vi "ListAllElementsDC.vi"(8 "error in (no error)":errorcluster, 11 "DataCollector in":refnum<class "DataCollector.lvclass">) -> (0 "error out":errorcluster, 1 "List of Fieldelements":string[](array[string]), 2 "Energy System Setup":string[][](table) caption="Result Set (from first statement with results)", 3 "DataCollector out":refnum<class "DataCollector.lvclass">)   [LabVIEW 2017, in "DataCollector.lvclass"]
uses:
  DataCollector.lvclass
  DataCollector.lvclass/DataCollector.ctl
  <vilib>/drjdpowell/SQLite Library/SQL Connection/Execute SQL.vi
  <vilib>/drjdpowell/SQLite Library/SQLite.lvlib
  <vilib>/drjdpowell/SQLite Library/SQL Connection/Connection.lvclass
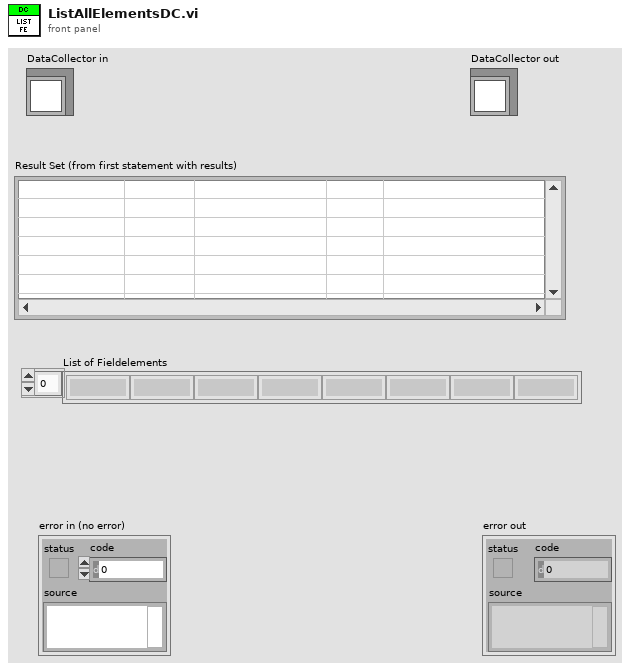
[diagram p1: front panel]
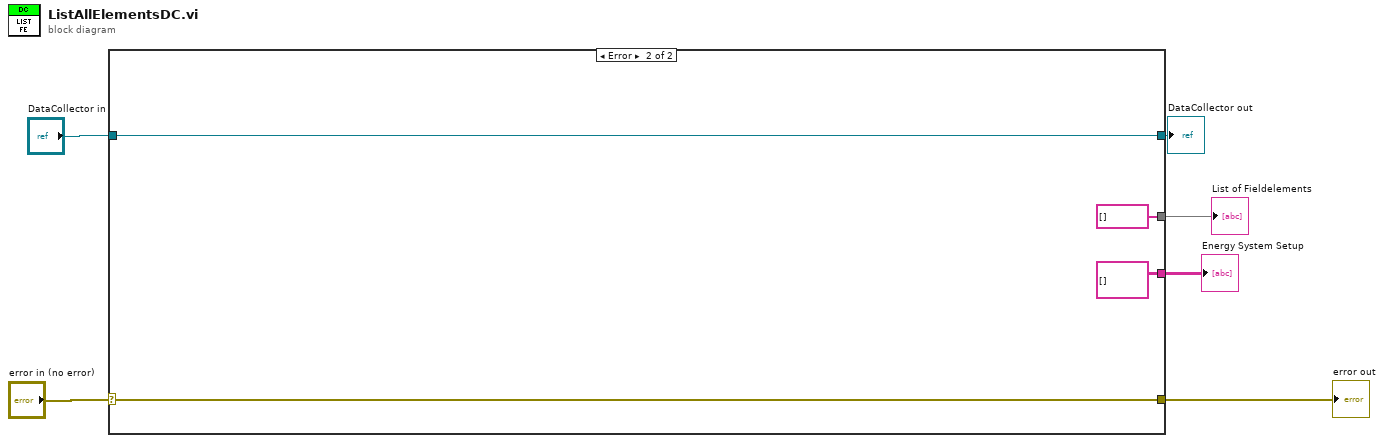
[diagram p0: block diagram]
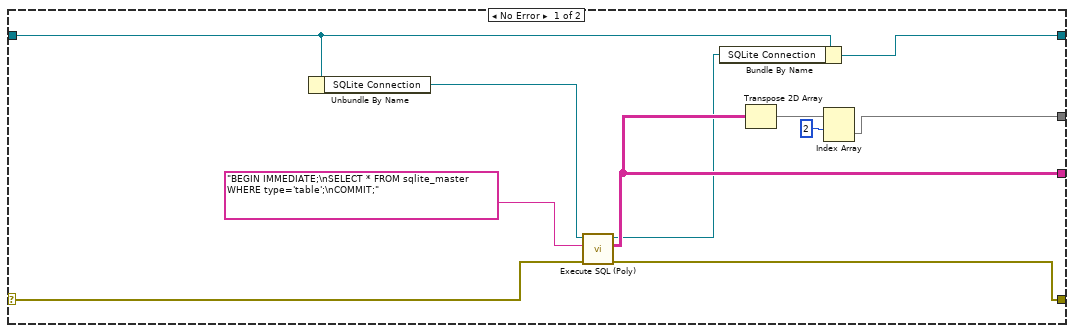
[diagram p2: hidden frame]
diagram:
  n1 = case shown="Error" "error in (no error)" {
    selector: "error in (no error)" -> [w12 w21]
    tunnel: [w11 w21] -> w5
    tunnel: [w9 w20] -> w3
    tunnel: "DataCollector in" -> [w10 w20]
    tunnel: [w15 string[][] [] ("Result Set")] -> w2
    tunnel: [w14 string[] []] -> w1
    frame No Error {
      n2 = Unbundle By Name(w10) -> ("SQLite Connection"=w8:refnum<class "Connection.lvclass">)
      n3 = call-poly <vilib>:"Execute SQL (Poly).vi"("error in (no error)"=w12, "SQL"="BEGIN IMMEDIATE;\nSELECT * FROM sqlite_master WHERE type='table';\nCOMMIT;" ("String"), "SQLite Connection in"=w8) -> ("error out"=w11:errorcluster, "Result Set"=w15:string[][], "SQLite Connection out"=w7:refnum<class "Connection.lvclass">)  [unwired: 5 in, 1 out]
      n4 = Bundle By Name(cluster=w10, "SQLite Connection"=w7) -> (w9:refnum<class "DataCollector.lvclass">)
      n5 = Transpose 2D Array(2D array=w15) -> (transposed array=w17:string[][])
      n6 = Index Array(array=w17, index (row)=2 ("Index")) -> (element=w14:string[])  [unwired: 1 in]
    }
    frame Error {
    }
  }
  "error out" <- w5
  "DataCollector out" <- w3
  "Energy System Setup" <- w2
  "List of Fieldelements" <- w1
